vi "VisaSendCmd.vi"(8 "error in (no error)":errorcluster, 9 "VISA resource name":refnum<visa-resource-name>, 11 "Msg to send":string) -> (0 "error out":errorcluster, 3 "VISA resource output":refnum<visa-resource-name>)   [LabVIEW 2021]
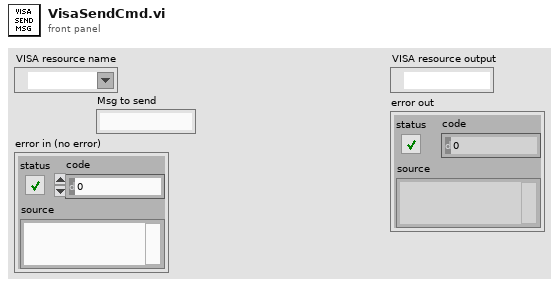
[diagram p1: front panel]
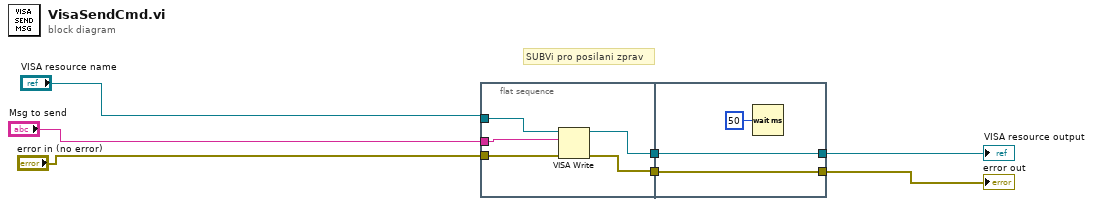
[diagram p0: block diagram]
diagram:
  # "SUBVi pro posilani zprav"
  n1 = flat-sequence {
    tunnel: "VISA resource name" -> [w12]
    tunnel: "error in (no error)" -> [w11]
    tunnel: "Msg to send" -> [w10]
    tunnel: [w9] -> w4
    tunnel: [w8] -> w3
    tunnel: [w15] -> w2
    tunnel: w4 -> [w15]
    tunnel: w3 -> [w14]
    tunnel: [w14] -> w1
    frame #0 {
      n2 = VISA Write(VISA resource name=w12, write buffer=w10, error in (no error)=w11) -> (VISA resource name out=w9:refnum<visa-resource-name>, error out=w8:errorcluster)  [unwired: 1 out]
    }
    frame #1 {
      n3 = Wait (ms)(milliseconds to wait=u32 50) -> ()  [unwired: 1 out]
    }
  }
  "VISA resource output" <- w2
  "error out" <- w1
